vi "Benchmark exprParser_parse_and_eval.vi"(8 "error in (no error)":errorcluster, 10 "Iterations":i32, 11 "Expression":string) -> (0 "error out":errorcluster, 2 "x":dbl[](array[numeric]), 3 "y":dbl[](array[numeric]), 5 "dt average":dbl)   [LabVIEW 2015]
uses:
  <vilib>/gmath/NI_Gmath.lvlib
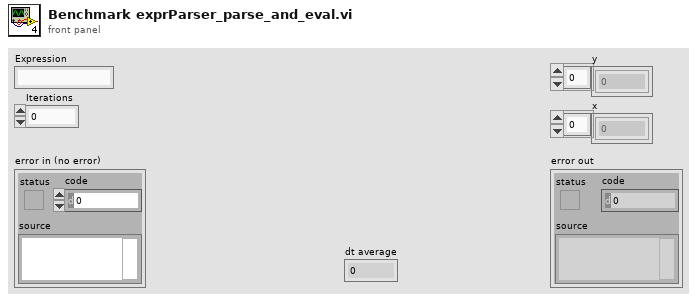
[diagram p1: front panel]
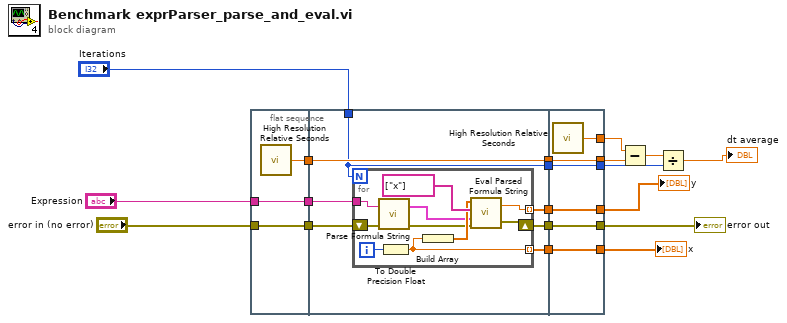
[diagram p0: block diagram]
diagram:
  n1 = flat-sequence {
    tunnel: "error in (no error)" -> [w21]
    tunnel: "Expression" -> [w22]
    tunnel: [w22] -> w17
    tunnel: [w21] -> w16
    tunnel: [w20] -> w11
    tunnel: w17 -> [w24]
    tunnel: w16 -> [w29]
    tunnel: [w28] -> w15
    tunnel: [w27] -> w14
    tunnel: [w26] -> w13
    tunnel: [w25] -> w12
    tunnel: w11 -> [w25]
    tunnel: "Iterations" -> [w23]
    tunnel: [w23] -> w5
    tunnel: [w43] -> w18
    tunnel: [w44] -> w19
    tunnel: [w45] -> w7
    tunnel: w15 -> [w45]
    tunnel: w14 -> [w44]
    tunnel: w13 -> [w43]
    tunnel: [w42] -> w9
    tunnel: w12 -> [w42]
    tunnel: [w41] -> w10
    tunnel: w5 -> [w40]
    tunnel: [w40] -> w4
    frame #0 {
      n2 = call <vilib>:"High Resolution Relative Seconds.vi"() -> ("relative seconds"=w20:dbl)
    }
    frame #1 {
      n3 = for {
        N: w23 -> [_]
        shift-right: [w34] -> w28
        shift-left: w29 -> [w32]
        tunnel: [w35] -> w27 mode=indexing
        tunnel: [w37] -> w26 mode=indexing
        tunnel: w24 -> [w33]
        i -> [w39]
        n4 = call <vilib>:"Parse Formula String.vi"("error in (no error)"=w32, "formula"=w33) -> ("error out"=w31:errorcluster, "Parsed Formula"=w30:cluster{"Table":i32[][], "Y Values":dbl[]})
        n5 = To Double Precision Float(number=w39) -> (double precision float=w37:dbl)
        n6 = Build Array(w37) -> (w36:dbl[])
        n7 = call <vilib>:"Eval Parsed Formula String.vi"("error in (no error)"=w31, "Parsed Formula"=w30, "Variables"=string[] ["x"], "X Values"=w36) -> ("error out"=w34:errorcluster, "y value"=w35:dbl)
      }
    }
    frame #2 {
      n8 = call <vilib>:"High Resolution Relative Seconds.vi"() -> ("relative seconds"=w41:dbl)
    }
  }
  n9 = Subtract(x=w10, y=w9) -> (x-y=w6:dbl)
  n10 = Divide(x=w6, y=w4) -> (x/y=→"dt average":dbl)
  "y" <- w19
  "x" <- w18
  "error out" <- w7
